vi "approxEqualDBL.vi"(1 "tol (1e-5)":dbl=1e-05 format="%#_13g", 2 "in2":dbl format="%#_13g", 3 "in1":dbl format="%#_13g") -> (0 "approximatelyEqual?":bool)   [LabVIEW 2015]
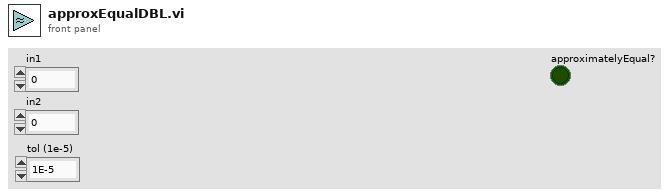
[diagram p1: front panel]
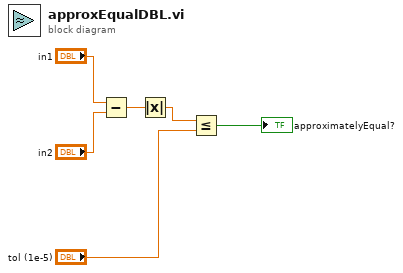
[diagram p0: block diagram]
diagram:
  n1 = Subtract(x="in1", y="in2") -> (x-y=w4:dbl)
  n2 = Absolute Value(x=w4) -> (abs(x)=w3:dbl)
  n3 = Less Or Equal?(x=w3, y="tol (1e-5)") -> (x <= y?=→"approximatelyEqual?":bool)
